vi "add channel to scan engine configuration.vi"(8 "error in":errorcluster, 10 "channel":refnum<class "TBM channel.lvclass">, 11 "Scan Engine configuration in":refnum<class "Scan Engine configuration.lvclass">) -> (0 "error out":errorcluster, 3 "Scan Engine configuration out":refnum<class "Scan Engine configuration.lvclass">)   [LabVIEW 2013, in "Scan Engine configuration.lvclass"]
uses:
  Scan Engine configuration.lvclass
  <vilib>/NI/Tag Bus Module Framework/channel/TBM channel.lvclass
  <vilib>/NI/Tag Bus/tag/tag descriptor.lvclass/tag descriptor.ctl
  Scan Engine configuration.lvclass/Scan Engine configuration.ctl
  <vilib>/NI/Tag Bus/tag/read tag name.vi
  <vilib>/NI/Tag Bus/tag/tag descriptor.lvclass
  <vilib>/NI/Configuration Framework/NISE_CEF_TreeControl.lvlib
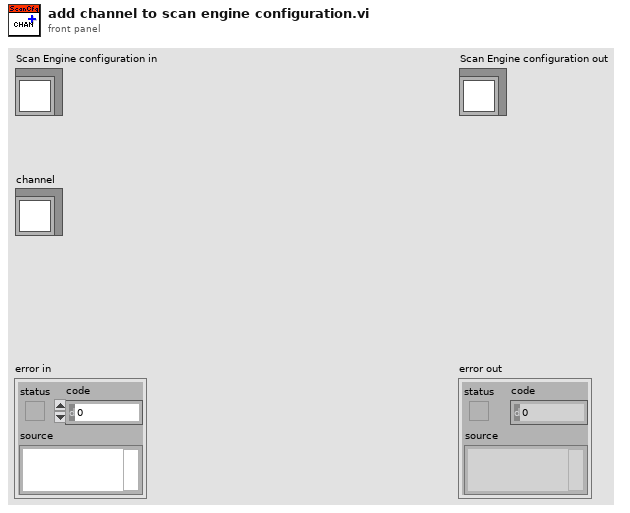
[diagram p1: front panel]
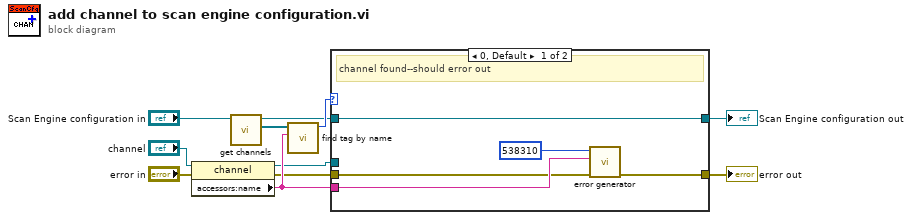
[diagram p0: block diagram]
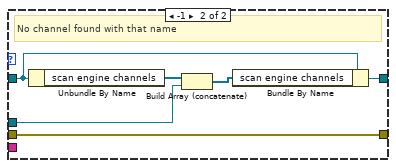
[diagram p2: hidden frame]
diagram:
  n1 = property class="channel"(reference="channel", error in="error in") -> (reference out=w7:refnum<class "TBM channel.lvclass">, error out=w6:errorcluster, "accessors:name"=w9:string)
  n2 = call-dynamic "get channels.vi"("module configuration in"="Scan Engine configuration in") -> ("channels"=w11:refnum<class "TBM channel.lvclass">[], "module configuration out"=w8:refnum<class "Scan Engine configuration.lvclass">)  [unwired: 9 in]
  n3 = call <vilib>:"find tag by name.vi"("name"=w9, "tags in"=w11) -> ("index"=w10:i32)  [unwired: 9 in]
  n4 = case shown="0, Default" w10 {
    tunnel: [w16 w22] -> w1
    tunnel: w9 -> [w14 _]
    tunnel: w6 -> [w13 w22]
    tunnel: w8 -> [w12 w20]
    tunnel: w7 -> [_ w21]
    tunnel: [w12 w17] -> w2
    frame 0, Default {
      # "channel found--should error out"
      n5 = call <vilib>:"error generator.vi"("error in"=w13, "append error message"=w14, "error code (0)"=538310) -> ("error out"=w16:errorcluster)  [unwired: 6 in]
    }
    frame -1 {
      # "No channel found with that name"
      n6 = Unbundle By Name(w20) -> ("scan engine channels"=w18:refnum<class "TBM channel.lvclass">[])
      n7 = Build Array (concatenate)(w18, w21) -> (w19:refnum<class "TBM channel.lvclass">[])
      n8 = Bundle By Name(cluster=w20, "scan engine channels"=w19) -> (w17:refnum<class "Scan Engine configuration.lvclass">)
    }
  }
  "error out" <- w1
  "Scan Engine configuration out" <- w2
